vi "delete.vi"(8 "error in (no error)":errorcluster, 11 "DoublyNodeRef in":refnum<class "DoublyNodeRef.lvclass">) -> (0 "error out":errorcluster)   [LabVIEW 2021, in "DoublyNodeRef.lvclass"]
uses:
  DoublyNodeRef.lvclass
  DoublyNodeRef.lvclass/DoublyNodeRef.ctl
  IDoublyNode/IDoublyNode.lvclass
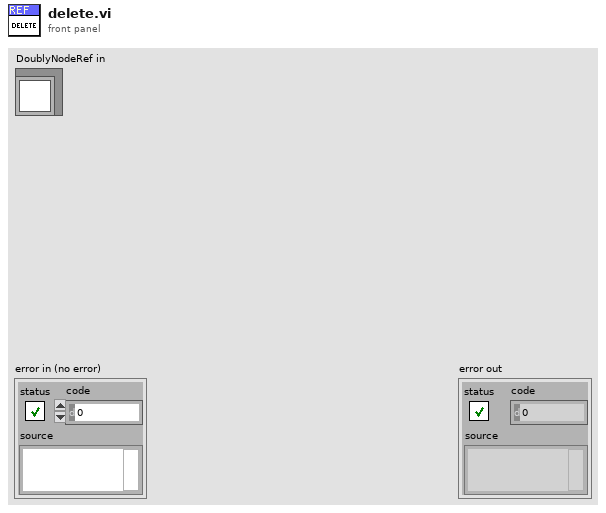
[diagram p1: front panel]
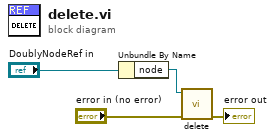
[diagram p0: block diagram]
diagram:
  n1 = Unbundle By Name("DoublyNodeRef in") -> ("node"=w3:refnum<data-value>)
  n2 = call "delete.vi"("error in (no error)"="error in (no error)", "node ref"=w3) -> ("error out"=→"error out":errorcluster)  [unwired: 9 in]
